vi "Reset.vi"(8 "error in (no error)":errorcluster, 11 "Proto Tag in":refnum<class "packed.lvclass">) -> (0 "error out":errorcluster, 3 "Proto Tag out":refnum<class "packed.lvclass">)   [LabVIEW 2020, in "Protobuf RAW.lvlib" / "packed.lvclass"]
uses:
  packed.lvclass
  Scalar Encoder/Scalar Type.lvclass
  packed.lvclass/packed.ctl
  Proto Type Common/Proto Type Common.lvclass
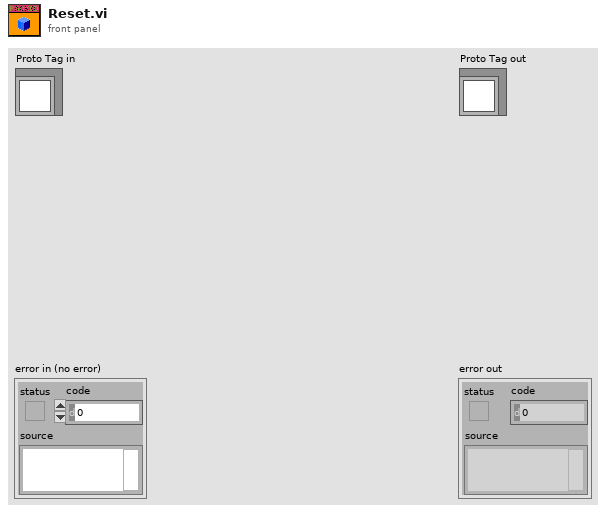
[diagram p1: front panel]
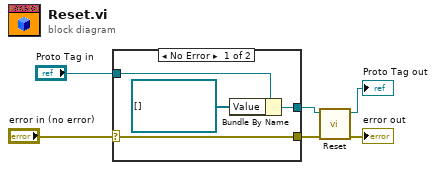
[diagram p0: block diagram]
diagram:
  n1 = case shown="No Error" "error in (no error)" {
    selector: "error in (no error)" -> [w8 w12]
    tunnel: "Proto Tag in" -> [w10 w11]
    tunnel: [w7 w11] -> w2
    tunnel: [w8 w12] -> w4
    frame No Error {
      n2 = Bundle By Name(cluster=w10, "Value"=refnum<class "Scalar Type.lvclass">[] []) -> (w7:refnum<class "packed.lvclass">)
    }
    frame Error {
    }
  }
  n3 = call-parent "Reset.vi"("error in (no error)"=w4, "Proto Type Common in"=w2) -> ("error out"=→"error out":errorcluster, "Proto Type Common out"=→"Proto Tag out":refnum<class "packed.lvclass">)  [unwired: 8 in]
